vi "Halvorsen_3DGraph.vi"() -> ()   [LabVIEW 2016]
uses:
  <vilib>/Native 3D Graph/xcontrol/3DPC_SurfacePlot.xctl
  <vilib>/Native 3D Graph/classes/Line/Line.lvclass
panel:
  in  "b":dbl[](array[numeric])=[0.1, 0.1, 0.1]
  out "Waveform Graph":dbl[][](graph)
  in  "Method":u16(ring) items=["ECD", "Euler", "EMP", "MEMP", "SEMP", "SIMP", "LIMP", "IEuler", "IMP"]
  in  "Hmax":dbl=1.0
  in  "Шаг h, с":dbl=0.01
  in  "Hmin":dbl=0.001
  in  "k":i32=4
  in  "tolerance":dbl=1e-17
  out "3D Graph (Error)":refnum<class "Base Datatype.lvclass">[](xcontrol)
  out "3D Graph (Solution)":refnum<class "Base Datatype.lvclass">[](xcontrol)
  in  "Время, с":dbl=30.0
  in  "Initial Conditions":dbl[](array[numeric])=[1.0, 0.0, 1.0]
  # "0 ECD1\n1 Euler\n2 Euler-Cromer\n3 EMP\n4 MEMP\n5 SEMP\n6 MSEMP\n7 SIMP\n8 MSIMP\n9 LIMP\n10 MLIMP\n11 MECD1"
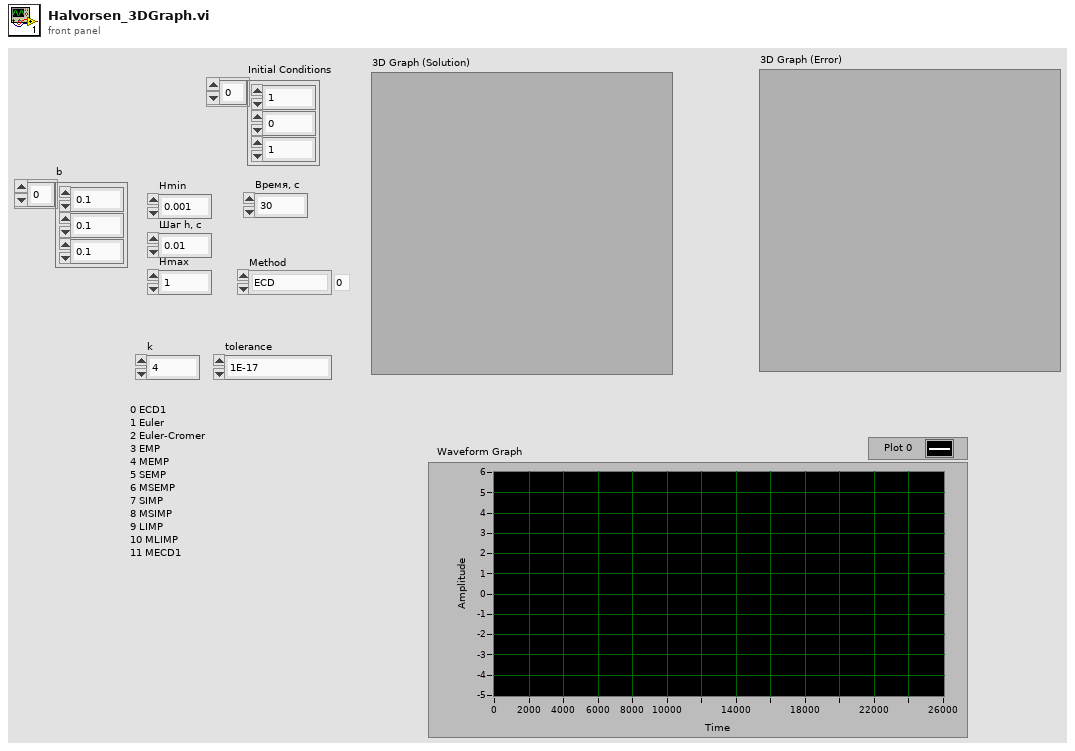
[diagram p1: front panel]
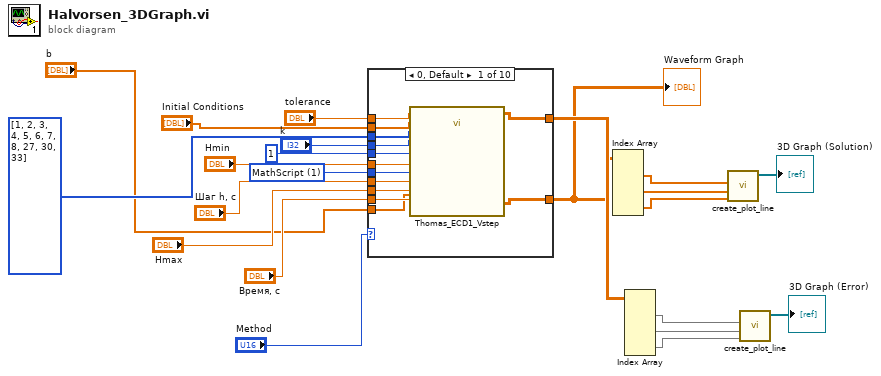
[diagram p0: block diagram]
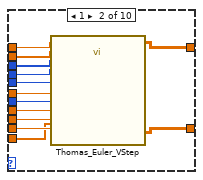
[diagram p2: hidden frame]
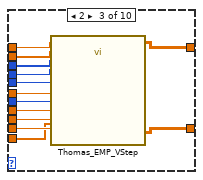
[diagram p3: hidden frame]
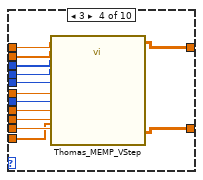
[diagram p4: hidden frame]
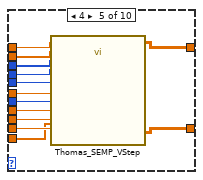
[diagram p5: hidden frame]
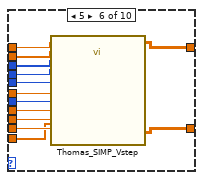
[diagram p6: hidden frame]
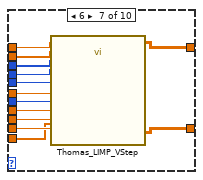
[diagram p7: hidden frame]
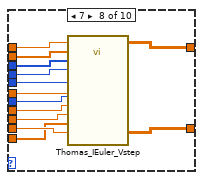
[diagram p8: hidden frame]
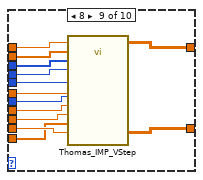
[diagram p9: hidden frame]
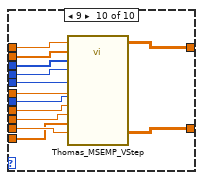
[diagram p10: hidden frame]
diagram:
  w8 = u16 1 items=["FNode", "MathScript", "ECD8 Arrays", "ECD8 Fnode", "ECD8 FnodeDiv", "FNode123"] ("Ext.Type")
  n1 = case shown="0, Default" "Method" {
    tunnel: [w35 w48 w61 w74 w87 w100 w113 w126 w139 w152] -> w2
    tunnel: [w34 w47 w60 w73 w86 w99 w112 w125 w138 w151] -> w3
    tunnel: "Initial Conditions" -> [w33 w46 w59 w72 w85 w98 w111 w124 w137 w150]
    tunnel: "tolerance" -> [w32 w45 w58 w71 w84 w97 w110 w123 w136 w149]
    tunnel: i32[] [1, 2, 3, 4, 5, 6, 7, 8, 27, 30, 33] ("n") -> [w31 w44 w57 w70 w83 w96 w109 w122 w135 w148]
    tunnel: "k" -> [w30 w43 w56 w69 w82 w95 w108 w121 w134 w147]
    tunnel: 1 ("Multiplier") -> [w29 w42 w55 w68 w81 w94 w107 w120 w133 w146]
    tunnel: "Hmin" -> [w28 w41 w54 w67 w80 w93 w106 w119 w132 w145]
    tunnel: w8 -> [w27 w40 w53 w66 w79 w92 w105 w118 w131 w144]
    tunnel: "Шаг h, с" -> [w26 w39 w52 w65 w78 w91 w104 w117 w130 w143]
    tunnel: "Hmax" -> [w25 w38 w51 w64 w77 w90 w103 w116 w129 w142]
    tunnel: "Время, с" -> [w24 w37 w50 w63 w76 w89 w102 w115 w128 w141]
    tunnel: "b" -> [w23 w36 w49 w62 w75 w88 w101 w114 w127 w140]
    frame 0, Default {
      n2 = call "Thomas_ECD1_Vstep.vi"("tolerance"=w32, "Время, с"=w24, "b"=w23, "Hmax"=w25, "Шаг h, с"=w26, "Initial Conditions"=w33, "n"=w31, "Ext.Type"=w27, "k"=w30, "Multiplier"=w29, "Hmin"=w28) -> ("Real Error"=w34:dbl[][], "Output_Signal"=w35:dbl[][])  [unwired: 3 in]
    }
    frame 1 {
      n3 = call "Thomas_Euler_VStep.vi"("tolerance"=w45, "Время, с"=w37, "b"=w36, "Hmax"=w38, "Шаг h, с"=w39, "Initial Conditions"=w46, "n"=w44, "Ext.Type"=w40, "k"=w43, "Multiplier"=w42, "Hmin"=w41) -> ("Real Error"=w47:dbl[][], "Output_Signal"=w48:dbl[][])  [unwired: 3 in]
    }
    frame 2 {
      n4 = call "Thomas_EMP_VStep.vi"("tolerance"=w58, "Время, с"=w50, "Parameter"=w49, "Hmax"=w51, "Шаг h, с"=w52, "Initial Conditions"=w59, "n"=w57, "Ext.Type"=w53, "k"=w56, "Multiplier"=w55, "Hmin"=w54) -> ("Real Error"=w60:dbl[][], "Output Signal"=w61:dbl[][])  [unwired: 3 in]
    }
    frame 3 {
      n5 = call "Thomas_MEMP_VStep.vi"("tolerance"=w71, "Время, с"=w63, "Parameter"=w62, "Hmax"=w64, "Шаг h, с"=w65, "Initial Conditions"=w72, "n"=w70, "Error Analysis"=w66, "k"=w69, "Multiplier"=w68, "Hmin"=w67) -> ("Real Error"=w73:dbl[][], "Output Signal"=w74:dbl[][])  [unwired: 3 in]
    }
    frame 4 {
      n6 = call "Thomas_SEMP_VStep.vi"("tolerance"=w84, "Время, с"=w76, "Parameter"=w75, "Hmax"=w77, "Шаг h, с"=w78, "Initial Conditions"=w85, "n"=w83, "Ext.Type"=w79, "k"=w82, "Multiplier"=w81, "Hmin"=w80) -> ("Real Error"=w86:dbl[][], "Output Signal"=w87:dbl[][])  [unwired: 3 in]
    }
    frame 5 {
      n7 = call "Thomas_SIMP_Vstep.vi"("tolerance"=w97, "Время, с"=w89, "Parameters"=w88, "Hmax"=w90, "Шаг h, с"=w91, "Initial Conditions"=w98, "n"=w96, "Ext.Type"=w92, "k"=w95, "Multiplier"=w94, "Hmin"=w93) -> ("Real Error"=w99:dbl[][], "Output_Signal"=w100:dbl[][])  [unwired: 3 in]
    }
    frame 6 {
      n8 = call "Thomas_LIMP_VStep.vi"("tolerance"=w110, "Время, с"=w102, "Parameters"=w101, "Hmax"=w103, "Шаг h, с"=w104, "Initial Conditions"=w111, "n"=w109, "Ext.Type"=w105, "k"=w108, "Multiplier"=w107, "Hmin"=w106) -> ("Real Error"=w112:dbl[][], "Output Signal"=w113:dbl[][])  [unwired: 3 in]
    }
    frame 7 {
      n9 = call "Thomas_IEuler_Vstep.vi"("tolerance"=w123, "Время, с"=w115, "b"=w114, "Hmax"=w116, "Шаг h, с"=w117, "Initial Conditions"=w124, "n"=w122, "Ext.Type"=w118, "k"=w121, "Multiplier"=w120, "Hmin"=w119) -> ("Real Error"=w125:dbl[][], "Output_Signal"=w126:dbl[][])  [unwired: 3 in]
    }
    frame 8 {
      n10 = call "Thomas_IMP_VStep.vi"("tolerance"=w136, "Время, с"=w128, "Parameters"=w127, "Hmax"=w129, "Шаг h, с"=w130, "Initial Conditions"=w137, "n"=w135, "Ext.Type"=w131, "k"=w134, "Multiplier"=w133, "Hmin"=w132) -> ("Real Error"=w138:dbl[][], "Output Signal"=w139:dbl[][])  [unwired: 3 in]
    }
    frame 9 {
      n11 = call "Thomas_MSEMP_VStep.vi"("tolerance"=w149, "Время, с"=w141, "Parameter"=w140, "Hmax"=w142, "Шаг h, с"=w143, "Initial Conditions"=w150, "n"=w148, "Error Analysis"=w144, "k"=w147, "Multiplier"=w146, "Hmin"=w145) -> ("Real Error"=w151:dbl[][], "Output Signal"=w152:dbl[][])  [unwired: 3 in]
    }
  }
  "Waveform Graph" <- w2
  n12 = Index Array(array=w2) -> (element #1=w21:dbl[], element #2=w20:dbl[], element #3=w19:dbl[])  [unwired: 6 in]
  n13 = Index Array(array=w3) -> (element #1=w16:dbl[], element #2=w17:dbl[], element #3=w18:dbl[])  [unwired: 6 in]
  n14 = call <vilib>:"create_plot_line.vi"("z vector"=w19, "y vector"=w20, "x vector"=w21) -> ("plots out"=→"3D Graph (Solution)":refnum<class "Base Datatype.lvclass">[])  [unwired: 2 in, 6 out]
  n15 = call <vilib>:"create_plot_line.vi"("z vector"=w18, "y vector"=w17, "x vector"=w16) -> ("plots out"=→"3D Graph (Error)":refnum<class "Base Datatype.lvclass">[])  [unwired: 2 in, 6 out]
